vi "Get Screw Data (SubVI).vi"(9 "Input Index":T2={"index"=210, "index 2"=213, "index 3"=216, "index 4"=219, "index 5"=222, "index 6"=225, "index 7"=228, "index 8"=260, "index 9"=180}, 11 "D Array":i16[](array[numeric])) -> (1 "玛脸捣DATA":T1)   [LabVIEW 2019]
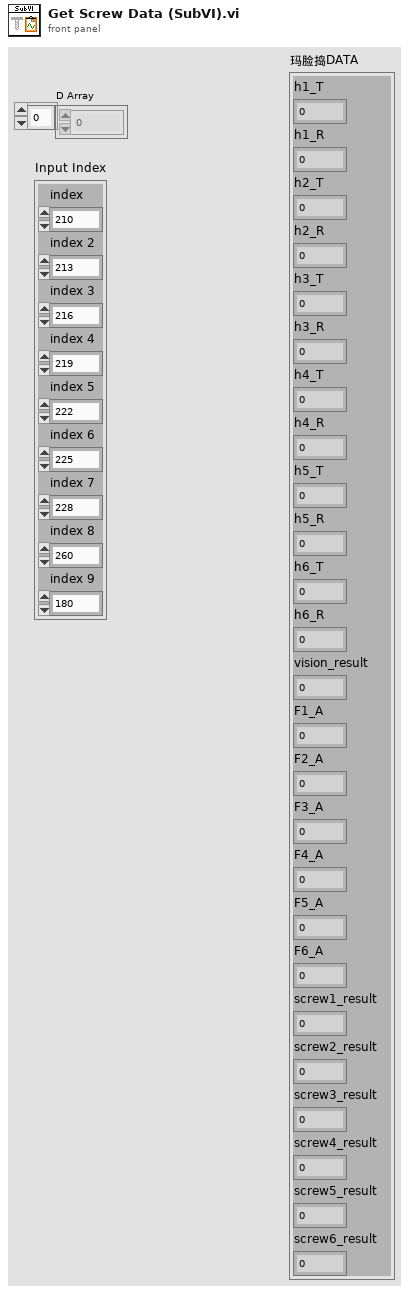
[diagram p1: front panel]
types:
  T1 = cluster{"h1_T":dbl, "h1_R":dbl, "h2_T":dbl, "h2_R":dbl, "h3_T":dbl, "h3_R":dbl, "h4_T":dbl, "h4_R":dbl, "h5_T":dbl, "h5_R":dbl, "h6_T":dbl, "h6_R":dbl, "vision_result":i32, "F1_A":dbl, "F2_A":dbl, "F3_A":dbl, "F4_A":dbl, "F5_A":dbl, "F6_A":dbl, "screw1_result":i32, "screw2_result":i32, "screw3_result":i32, "screw4_result":i32, "screw5_result":i32, "screw6_result":i32}
  T2 = cluster{"index":i32, "index 2":i32, "index 3":i32, "index 4":i32, "index 5":i32, "index 6":i32, "index 7":i32, "index 8":i32, "index 9":i32}
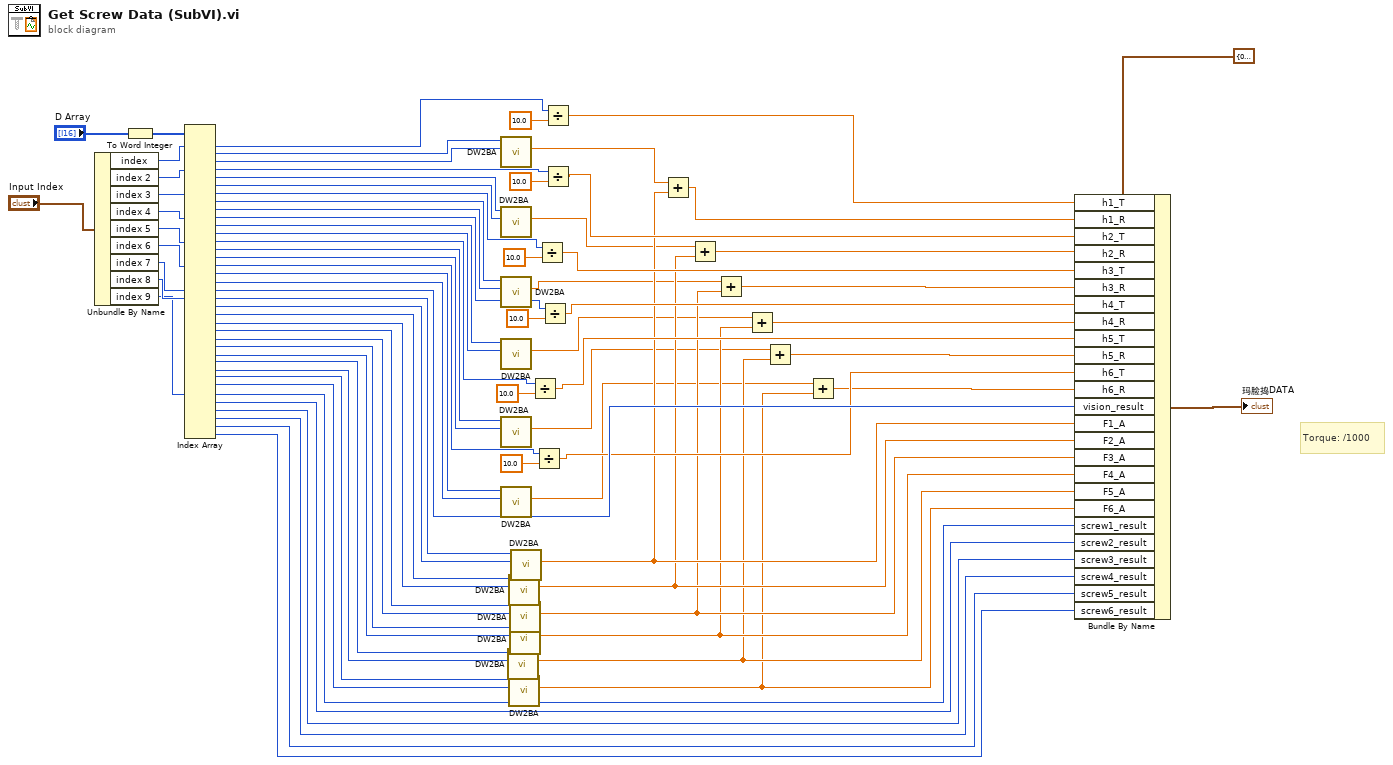
[diagram p0: block diagram]
diagram:
  # "Torque: /1000"
  n1 = Unbundle By Name("Input Index") -> ("index"=w67:i32, "index 2"=w66:i32, "index 3"=w65:i32, "index 4"=w64:i32, "index 5"=w63:i32, "index 6"=w62:i32, "index 7"=w61:i32, "index 8"=w39:i32, "index 9"=w7:i32)
  n2 = To Word Integer(number="D Array") -> (16bit integer=w68:i16[])
  n3 = Index Array(array=w68, index #1=w67, index #4=w66, index #7=w65, index #10=w64, index #13=w63, index #16=w62, index #19=w61, index #20=w39, index #32=w7) -> (element #1=w56:i16, element #2=w70:i16, element #3=w71:i16, element #4=w52:i16, element #5=w72:i16, element #6=w73:i16, element #7=w49:i16, element #8=w74:i16, element #9=w75:i16, element #10=w47:i16, element #11=w76:i16, element #12=w77:i16, element #13=w44:i16, element #14=w78:i16, element #15=w79:i16, element #16=w40:i16, element #17=w80:i16, element #18=w81:i16, element #19=w58:i16, element #20=w38:i16, element #21=w37:i16, element #22=w36:i16, element #23=w35:i16, element #24=w34:i16, element #25=w33:i16, element #26=w32:i16, element #27=w31:i16, element #28=w30:i16, element #29=w29:i16, element #30=w28:i16, element #31=w27:i16, element #32=w6:i16, element #33=w5:i16, element #34=w4:i16, element #35=w3:i16, element #36=w2:i16, element #37=w1:i16)  [unwired: 28 in]
  n4 = call "DW2BA.vi"("DW01"=w71, "DW00"=w70) -> ("圈數"=w26:dbl)  [unwired: 8 in, 1 out]
  n5 = call "DW2BA.vi"("DW01"=w73, "DW00"=w72) -> ("圈數"=w23:dbl)  [unwired: 8 in, 1 out]
  n6 = call "DW2BA.vi"("DW01"=w75, "DW00"=w74) -> ("圈數"=w20:dbl)  [unwired: 8 in, 1 out]
  n7 = call "DW2BA.vi"("DW01"=w77, "DW00"=w76) -> ("圈數"=w17:dbl)  [unwired: 8 in, 1 out]
  n8 = call "DW2BA.vi"("DW01"=w79, "DW00"=w78) -> ("圈數"=w14:dbl)  [unwired: 8 in, 1 out]
  n9 = call "DW2BA.vi"("DW01"=w81, "DW00"=w80) -> ("圈數"=w11:dbl)  [unwired: 8 in, 1 out]
  n10 = call "DW2BA.vi"("DW01"=w29, "DW00"=w30) -> ("圈數"=w12:dbl)  [unwired: 8 in, 1 out]
  n11 = call "DW2BA.vi"("DW01"=w35, "DW00"=w36) -> ("圈數"=w22:dbl)  [unwired: 8 in, 1 out]
  n12 = call "DW2BA.vi"("DW01"=w27, "DW00"=w28) -> ("圈數"=w9:dbl)  [unwired: 8 in, 1 out]
  n13 = call "DW2BA.vi"("DW01"=w33, "DW00"=w34) -> ("圈數"=w19:dbl)  [unwired: 8 in, 1 out]
  n14 = call "DW2BA.vi"("DW01"=w31, "DW00"=w32) -> ("圈數"=w15:dbl)  [unwired: 8 in, 1 out]
  n15 = call "DW2BA.vi"("DW01"=w37, "DW00"=w38) -> ("圈數"=w25:dbl)  [unwired: 8 in, 1 out]
  n16 = Divide(x=w44, y=10.0) -> (x/y=w43:dbl)
  n17 = Divide(x=w40, y=10.0) -> (x/y=w41:dbl)
  n18 = Divide(x=w49, y=10.0) -> (x/y=w50:dbl)
  n19 = Divide(x=w47, y=10.0) -> (x/y=w46:dbl)
  n20 = Divide(x=w56, y=10.0) -> (x/y=w55:dbl)
  n21 = Divide(x=w52, y=10.0) -> (x/y=w53:dbl)
  n22 = Add(x=w26, y=w25) -> (x+y=w24:dbl)
  n23 = Add(x=w23, y=w22) -> (x+y=w21:dbl)
  n24 = Add(x=w20, y=w19) -> (x+y=w18:dbl)
  n25 = Add(x=w17, y=w15) -> (x+y=w16:dbl)
  n26 = Add(x=w14, y=w12) -> (x+y=w13:dbl)
  n27 = Add(x=w11, y=w9) -> (x+y=w10:dbl)
  n28 = Bundle By Name(cluster=T1 {"h1_T"=0.0, "h1_R"=0.0, "h2_T"=0.0, "h2_R"=0.0, "h3_T"=0.0, "h3_R"=0.0, "h4_T"=0.0, "h4_R"=0.0, "h5_T"=0.0, "h5_R"=0.0, "h6_T"=0.0, "h6_R"=0.0, "vision_result"=0, "F1_A"=0.0, "F2_A"=0.0, "F3_A"=0.0, "F4_A"=0.0, "F5_A"=0.0, "F6_A"=0.0, "screw1_result"=0, "screw2_result"=0, "screw3_result"=0, "screw4_result"=0, "screw5_result"=0, "screw6_result"=0} ("玛脸捣DATA"), "h1_T"=w55, "h1_R"=w24, "h2_T"=w53, "h2_R"=w21, "h3_T"=w50, "h3_R"=w18, "h4_T"=w46, "h4_R"=w16, "h5_T"=w43, "h5_R"=w13, "h6_T"=w41, "h6_R"=w10, "vision_result"=w58, "F1_A"=w25, "F2_A"=w22, "F3_A"=w19, "F4_A"=w15, "F5_A"=w12, "F6_A"=w9, "screw1_result"=w6, "screw2_result"=w5, "screw3_result"=w4, "screw4_result"=w3, "screw5_result"=w2, "screw6_result"=w1) -> (→"玛脸捣DATA":T1)
